vi "Overwrite Item (inline).vi"(8 "error in (no error)":errorcluster, 9 "BetterTreeItem in":refnum<class "BetterItem.lvclass">, 10 "Item Index":i32, 11 "BetterHandle in":refnum<class "BetterHandle.lvclass">) -> (0 "error out":errorcluster, 3 "BetterHandle out":refnum<class "BetterHandle.lvclass">)   [LabVIEW 2020, in "BetterDragAndDrop.lvlib" / "BetterHandle.lvclass"]
uses:
  BetterHandle.lvclass
  BetterTreeItem/BetterItem.lvclass
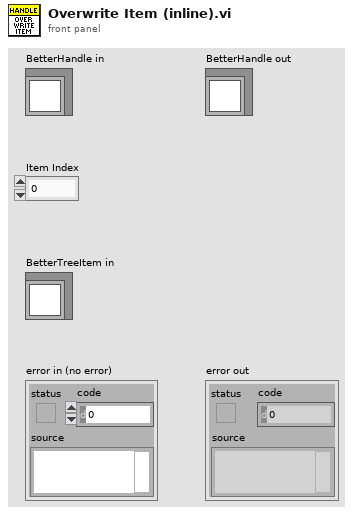
[diagram p1: front panel]
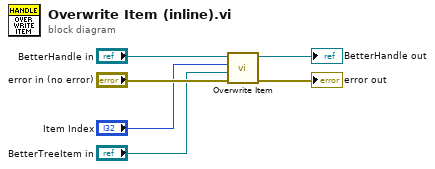
[diagram p0: block diagram]
diagram:
  n1 = call-dynamic "Overwrite Item.vi"("error in (no error)"="error in (no error)", "BetterTreeItem in"="BetterTreeItem in", "TreeItem Index"="Item Index", "BetterHandle in"="BetterHandle in") -> ("error out"=→"error out":errorcluster, "BetterHandle out"=→"BetterHandle out":refnum<class "BetterHandle.lvclass">)  [unwired: 6 in]
